vi "Open Motors.vi"(11 "PID Constants for Sparks":T6={"P Gain"=0.00035, "I Gain"=5e-07, "D Gain"=0.0, "F Gain"=0.0002, "I Zone"=0.0, "Min Output"=-1.0, "Max Output"=1.0}) -> (0 "error out":errorcluster, 3 "motors":cluster{"left master":T1, "right master":T1})   [LabVIEW 2019]
uses:
  <vilib>/Rock Robotics/WPI/MotorControl/WPI_MotorControlDeviceRef.ctl
  <vilib>/Rock Robotics/WPI/MotorControl/WPI_MotorControlType.ctl
  <vilib>/Rock Robotics/SystemInterfaces/DIO/FPGA_DIOPWMChannel.ctl
  <vilib>/Rock Robotics/WPI/PWM/WPI_PWMDeadband.ctl
  <vilib>/Rock Robotics/SystemInterfaces/DIO/FPGA_DIOChannel.ctl
  <vilib>/Rock Robotics/WPI/ThirdParty/REV Robotics/SPARK MAX/Typedef/Spark MAX Idle Mode.ctl
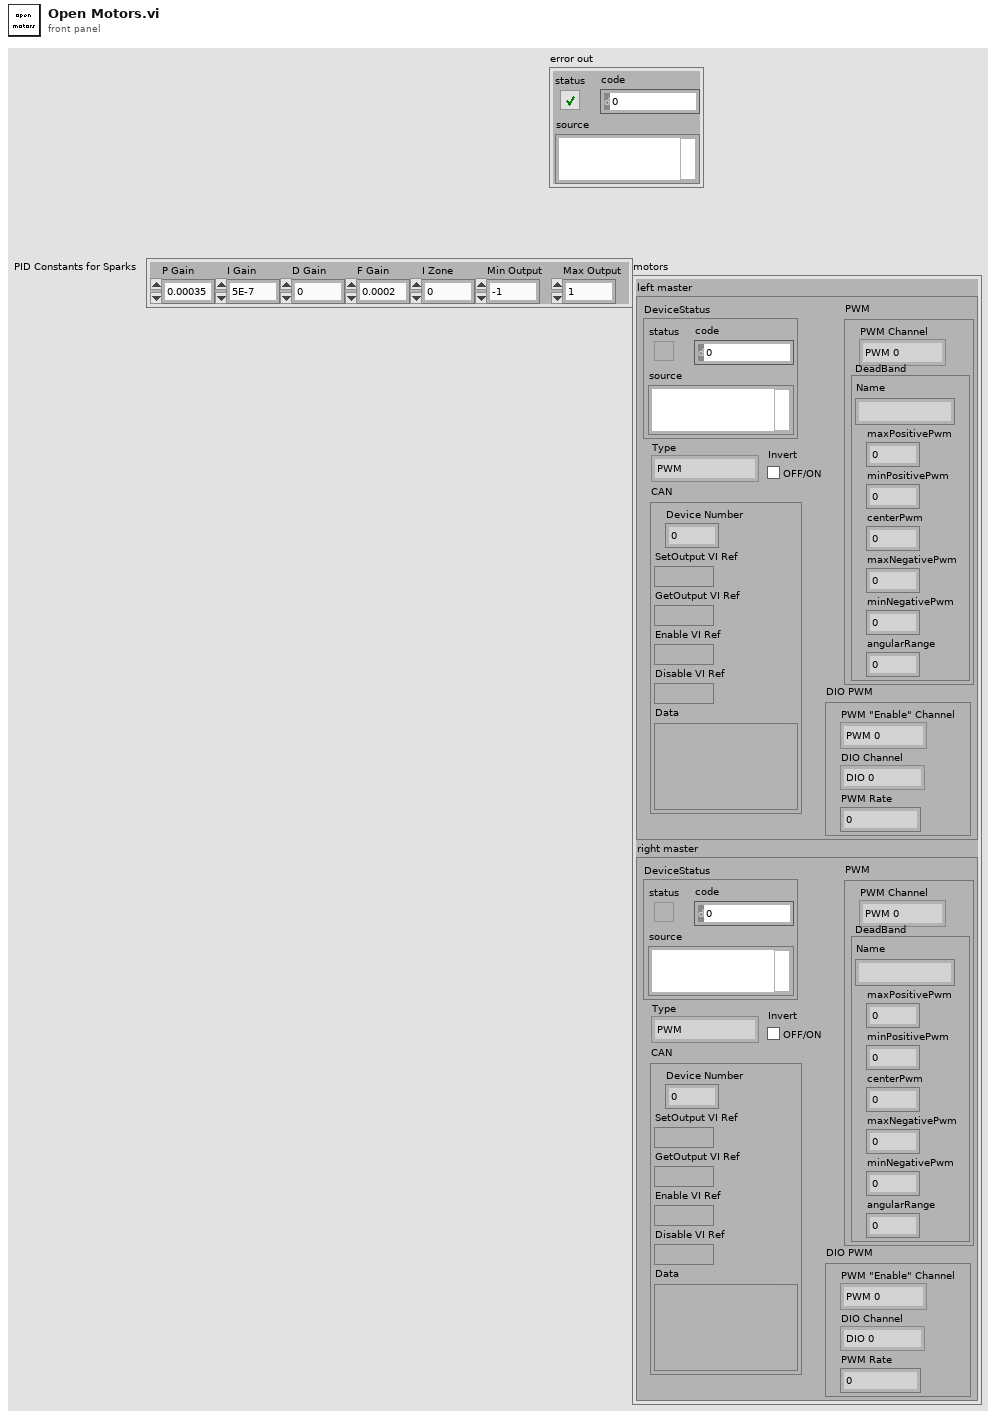
[diagram p1: front panel]
types:
  T1 = typedef "WPI_MotorControlDeviceRef.ctl" = cluster{"DeviceStatus":errorcluster, "Type":T2, "PWM":cluster{"PWM Channel":T3, "DeadBand":T4}, "CAN":cluster{"Device Number":u8, "SetOutput VI Ref":variant, "GetOutput VI Ref":variant, "Enable VI Ref":variant, "Disable VI Ref":variant, "Data":variant}, "Invert":bool, "DIO PWM":cluster{"PWM \"Enable\" Channel":T3, "DIOChannel":T5, "PWM Rate":dbl}}
  T2 = typedef "WPI_MotorControlType.ctl" = enum16{"PWM", "CAN", "DIO PWM"}
  T3 = typedef "FPGA_DIOPWMChannel.ctl" = enum8{"PWM 0", "PWM 1", "PWM 2", "PWM 3", "PWM 4", "PWM 5", "PWM 6", "PWM 7", "PWM 8", "PWM 9", "PWM MXP 0", "PWM MXP 1", "PWM MXP 2", "PWM MXP 3", "PWM MXP 4", "PWM MXP 5", "PWM MXP 6", "PWM MXP 7", "PWM MXP 8", "PWM MXP 9", "Invalid"}
  T4 = typedef "WPI_PWMDeadband.ctl" = cluster{"Name":string, "maxPositivePwm":i32, "minPositivePwm":i32, "centerPwm":i32, "maxNegativePwm":i32, "minNegativePwm":i32, "angularRange":u16}
  T5 = typedef "FPGA_DIOChannel.ctl" = enum8{"DIO 0", "DIO 1", "DIO 2", "DIO 3", "DIO 4", "DIO 5", "DIO 6", "DIO 7", "DIO 8", "DIO 9", "DIO MXP 0", "DIO MXP 1", "DIO MXP 2", "DIO MXP 3", "DIO MXP 4", "DIO MXP 5", "DIO MXP 6", "DIO MXP 7", "DIO MXP 8", "DIO MXP 9", "DIO MXP 10", "DIO MXP 11", "DIO MXP 12", "DIO MXP 13", "DIO MXP 14", "DIO MXP 15", "SPI Port CS1", "SPI Port CS2", "SPI Port CS3", "SPI Port MISO", "SPI Port MOSI", "Invalid"}
  T6 = cluster{"P Gain":dbl, "I Gain":dbl, "D Gain":dbl, "F Gain":dbl, "I Zone":dbl, "Min Output":dbl, "Max Output":dbl}
  T7 = typedef "Spark MAX Idle Mode.ctl" = enum16{"Coast", "Brake"}
  T8 = cluster{"MotorControlDeviceRef":T1, "MotorControlDeviceRef":T1}
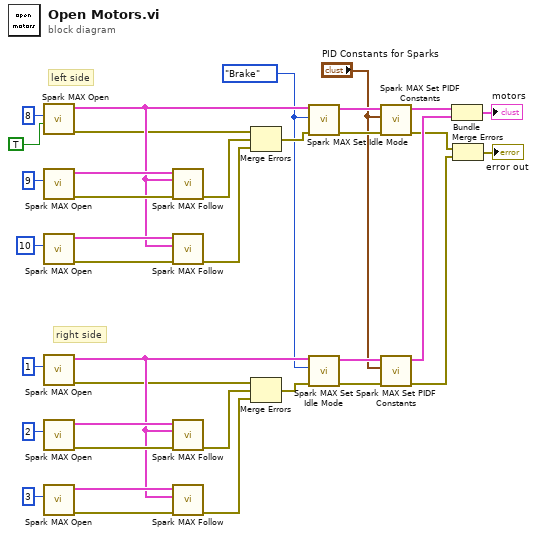
[diagram p0: block diagram]
diagram:
  w6 = Spark_MAX_Idle_Mode."Brake" ("Idle Mode")
  # "right side"
  # "left side"
  n1 = call <vilib>:"Spark MAX Open.vi"("Invert"=TRUE, "Device Number"=u8 8) -> ("error out"=w27:errorcluster, "MotorControlDeviceRef"=w30:T1)  [unwired: 8 in]
  n2 = call <vilib>:"Spark MAX Open.vi"("Device Number"=u8 9) -> ("error out"=w34:errorcluster, "MotorControlDeviceRef"=w32:T1)  [unwired: 9 in]
  n3 = call <vilib>:"Spark MAX Open.vi"("Device Number"=u8 10) -> ("error out"=w33:errorcluster, "MotorControlDeviceRef"=w31:T1)  [unwired: 9 in]
  n4 = call <vilib>:"Spark MAX Open.vi"("Device Number"=u8 1) -> ("error out"=w13:errorcluster, "MotorControlDeviceRef"=w16:T1)  [unwired: 9 in]
  n5 = call <vilib>:"Spark MAX Open.vi"("Device Number"=u8 2) -> ("error out"=w20:errorcluster, "MotorControlDeviceRef"=w18:T1)  [unwired: 9 in]
  n6 = call <vilib>:"Spark MAX Open.vi"("Device Number"=u8 3) -> ("error out"=w19:errorcluster, "MotorControlDeviceRef"=w17:T1)  [unwired: 9 in]
  n7 = call <vilib>:"Spark MAX Follow.vi"("error in (no error)"=w34, "Master Controller"=w30, "MotorControlDeviceRef"=w32) -> ("error out"=w29:errorcluster)  [unwired: 7 in, 1 out]
  n8 = call <vilib>:"Spark MAX Follow.vi"("error in (no error)"=w33, "Master Controller"=w30, "MotorControlDeviceRef"=w31) -> ("error out"=w28:errorcluster)  [unwired: 7 in, 1 out]
  n9 = call <vilib>:"Spark MAX Follow.vi"("error in (no error)"=w20, "Master Controller"=w16, "MotorControlDeviceRef"=w18) -> ("error out"=w15:errorcluster)  [unwired: 7 in, 1 out]
  n10 = call <vilib>:"Spark MAX Follow.vi"("error in (no error)"=w19, "Master Controller"=w16, "MotorControlDeviceRef"=w17) -> ("error out"=w14:errorcluster)  [unwired: 7 in, 1 out]
  n11 = Merge Errors(w27, w29, w28) -> (w26:errorcluster)
  n12 = Merge Errors(w13, w15, w14) -> (w12:errorcluster)
  n13 = call <vilib>:"Spark MAX Set Idle Mode.vi"("error in (no error)"=w26, "Idle Mode"=w6, "MotorControlDeviceRef in"=w30) -> ("error out"=w24:errorcluster, "MotorControlDeviceRef out"=w25:T1)  [unwired: 7 in]
  n14 = call <vilib>:"Spark MAX Set Idle Mode.vi"("error in (no error)"=w12, "Idle Mode"=w6, "MotorControlDeviceRef in"=w16) -> ("error out"=w10:errorcluster, "MotorControlDeviceRef out"=w11:T1)  [unwired: 7 in]
  n15 = call <vilib>:"Spark MAX Set PIDF Constants.vi"("error in"=w24, "PID Constants"="PID Constants for Sparks", "MotorControlDeviceRef"=w25) -> ("error out"=w5:errorcluster, "MotorControlDeviceRef"=w8:T1)  [unwired: 7 in]
  n16 = call <vilib>:"Spark MAX Set PIDF Constants.vi"("error in"=w10, "PID Constants"="PID Constants for Sparks", "MotorControlDeviceRef"=w11) -> ("error out"=w4:errorcluster, "MotorControlDeviceRef"=w7:T1)  [unwired: 7 in]
  n17 = Bundle("MotorControlDeviceRef"=w8, "MotorControlDeviceRef"=w7) -> (→"motors":T8)  [unwired: 1 in]
  n18 = Merge Errors(w5, w4) -> (→"error out":errorcluster)
